vi "set task timing.vi"(8 "error in (no error)":errorcluster, 11 "Waveform in":refnum<class "Waveform.lvclass">) -> (0 "error out":errorcluster, 3 "Waveform out":refnum<class "Waveform.lvclass">)   [LabVIEW 2012, in "Waveform.lvclass"]
uses:
  Waveform.lvclass
  Waveform.lvclass/Waveform.ctl
  <vilib>/DAQmx/configure/timing.llb/DAQmx Timing (Implicit).vi
  <vilib>/DAQmx/configure/timing.llb/DAQmx Timing (Sample Clock).vi
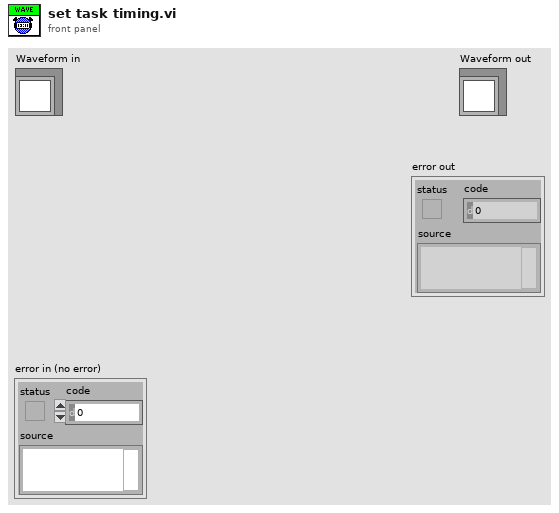
[diagram p1: front panel]
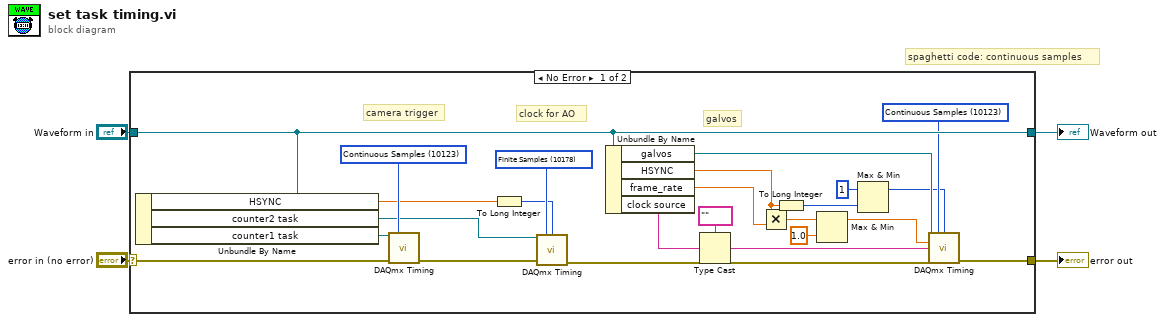
[diagram p0: block diagram]
diagram:
  # "spaghetti code: continuous samples"
  n1 = case shown="No Error" "error in (no error)" {
    selector: "error in (no error)" -> [w26 w30]
    tunnel: [w12 w30] -> w3
    tunnel: [w23 w29] -> w1
    tunnel: "Waveform in" -> [w23 w29]
    frame No Error {
      w18 = 10178 items=["Finite Samples"=10178, "Continuous Samples"=10123, "Hardware Timed Single Point"=12522] ("sample mode")
      w21 = 10123 items=["Finite Samples"=10178, "Continuous Samples"=10123, "Hardware Timed Single Point"=12522] ("sample mode")
      w28 = 10123 items=["Finite Samples"=10178, "Continuous Samples"=10123, "Hardware Timed Single Point"=12522] ("sample mode")
      # "galvos"
      # "camera trigger"
      # "clock for AO"
      n2 = Unbundle By Name(w23) -> ("HSYNC"=w16:dbl, "counter2 task"=w17:refnum<k21>, "counter1 task"=w27:refnum<k21>)
      n3 = call-poly <vilib>:"DAQmx Timing.vi"("task/channels in"=w27, "sample mode"=w28, "error in"=w26) -> ("error out"=w20:errorcluster)  [unwired: 11 in, 1 out]
      n4 = To Long Integer(number=w16) -> (32bit integer=w15:i32)
      n5 = call-poly <vilib>:"DAQmx Timing.vi"("task/channels in"=w17, "sample mode"=w18, "samples per channel"=w15, "error in"=w20) -> ("error out"=w19:errorcluster)  [unwired: 10 in, 1 out]
      n6 = Unbundle By Name(w23) -> ("galvos"=w22:refnum<k21>, "HSYNC"=w24:dbl, "frame_rate"=w25:dbl, "clock source"=w14:string)
      n7 = Type Cast(type=tag "" ("source"), x=w14) -> (*(type *) &x=w11:tag)
      n8 = Multiply(x=w24, y=w25) -> (x*y=w7:dbl)
      n9 = To Long Integer(number=w24) -> (32bit integer=w9:i32)
      n10 = Max & Min(x=w7, y=1.0) -> (max(x,y)=w6:dbl)  [unwired: 1 out]
      n11 = Max & Min(x=1, y=w9) -> (max(x,y)=w8:i32)  [unwired: 1 out]
      n12 = call-poly <vilib>:"DAQmx Timing.vi"("task/channels in"=w22, "sample mode"=w21, "samples per channel"=w8, "rate"=w6, "source"=w11, "error in"=w19) -> ("error out"=w12:errorcluster)  [unwired: 8 in, 1 out]
    }
    frame Error {
    }
  }
  "error out" <- w3
  "Waveform out" <- w1
